vi "Mod_OFDM_Examine_Configure_Data_Sources.vi"(0 "Configuration in":variant, 11 "error in":errorcluster) -> (4 "Configuration out":variant, 15 "error out":errorcluster)   [LabVIEW 2010]
doc: "The VI performs three functions:\n\n1) Examine pool of data sources that have been configured.\n\n2) Add/Edit the current pool of Data sources. By default four Data sources are pre-configured.\n\n3) To store the current pool of data sources in the configuration Variant"
uses:
  Polymorphic_Sub_VI's/Mod_OFDM_Get_Data_Sources.vi
  Polymorphic_Sub_VI's/Mod_OFDM_Set_Data_Source.vi
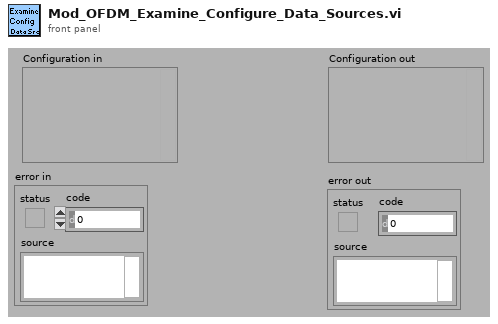
[diagram p1: front panel]
types:
  T1 = typedef "Pool of Data Source Control.ctl" = cluster{"mode (PN)":enum16{"PN", "pattern", "user"}, "PN sequence order (9)":i32, "Invert Output Bits":enum16{"No", "Yes"}, "Register Initial State ":u32, "User base bit pattern":i8[], "base bit pattern (00001111)":enum16{"0", "1", "01", "0011", "00001111"}, "Reset to Initial State":enum16{"Every OFDM Frame", "Every OFDM Symbol", "Every Sub Carrier"}}[]
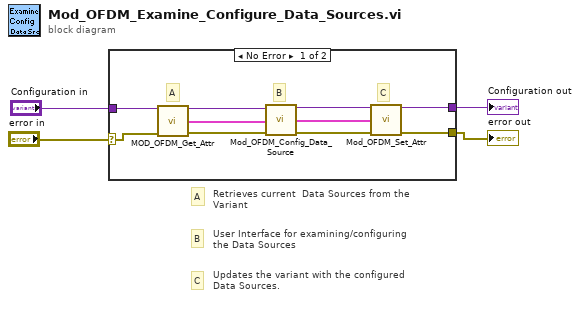
[diagram p0: block diagram]
diagram:
  # "Updates the variant with the configured Data Sources."
  # "User Interface for examining/configuring the Data Sources"
  # "Retrieves current  Data Sources from the Variant"
  # "A"
  # "C"
  # "B"
  n1 = case shown="No Error" "error in" {
    selector: "error in" -> [w10 w15]
    tunnel: "Configuration in" -> [w14 _]
    tunnel: [w11 _] -> w3
    tunnel: [w9 w15] -> w1
    frame No Error {
      # "C"
      # "B"
      # "A"
      n2 = call-poly "MOD_OFDM_Get_Attr.vi"("Configuration in"=w14, "error in"=w10) -> ("Configuration out"=w8:variant, "Pool of Data Sources"=w6:T1, "error out"=w13:errorcluster)  [unwired: 7 in, 4 out]
      n3 = call "Mod_OFDM_Config_Data_Source.vi"("Configuration in"=w8, "Pool of Data Sources"=w6, "error in"=w13) -> ("Configuration out"=w7:variant, "Pool of Data Sources"=w5:T1, "error out"=w12:errorcluster)  [unwired: 10 in]
      n4 = call-poly "Mod_OFDM_Set_Attr.vi"("Configuration in"=w7, "Pool of Data Sources"=w5, "error in"=w12) -> ("Configuration out"=w11:variant, "error out"=w9:errorcluster)  [unwired: 11 in]
    }
    frame Error {
    }
  }
  "Configuration out" <- w3
  "error out" <- w1
